vi "Render.vi"(8 "error in":errorcluster, 10 "Renderer in":refnum<class "Renderer.lvclass">, 11 "Dqmh Event in":refnum<class "Dqmh Event.lvclass">) -> (0 "error out":errorcluster, 3 "Sections out":refnum<class "Section.lvclass">[](array[class]))   [LabVIEW 2021, in "TAF Proj Document Type.lvlib" / "Dqmh Event.lvclass"]
uses:
  <vilib>/Wovalab/AntiDoc/Document Type/Add-ons/LabVIEW TAF Project/Dqmh Event/Dqmh Event.lvclass
  C:/Program Files (x86)/National Instruments/LabVIEW 2021/vi.lib/Wovalab/AntiDoc/Document Type/Add-ons/LabVIEW TAF Project/Vi/Vi.lvclass
  C:/Program Files (x86)/National Instruments/LabVIEW 2021/vi.lib/Wovalab/AntiDoc/Bloc/Bloc.lvclass
  <vilib>/Wovalab/AntiDoc/Renderer/Renderer.lvclass
  <vilib>/Wovalab/AsciiDoc for LabVIEW/Section/Section.lvclass
  <vilib>/Wovalab/AntiDoc/Document Type/Add-ons/LabVIEW TAF Project/Dqmh Event/Dqmh Event.lvclass/Dqmh Event.ctl
  <vilib>/Wovalab/AntiDoc/Document Type/Add-ons/LabVIEW TAF Project/Vi/Vi.lvclass/Vi.ctl
  <vilib>/Wovalab/AntiDoc/Bloc/Bloc.lvclass/Bloc.ctl
  <vilib>/Wovalab/AntiDoc/Renderer/Renderer.lvclass/Renderer.ctl
  <vilib>/Wovalab/AntiDoc/Renderer/Read Image Folder Path.vi
  <vilib>/Wovalab/AntiDoc/Document Type/Add-ons/LabVIEW TAF Project/Dqmh Event/Read Event Type.vi
  <vilib>/Wovalab/AntiDoc/Document Type/Add-ons/LabVIEW TAF Project/Vi/Read Conpane Image.vi
  <vilib>/Wovalab/AntiDoc/Bloc/Read Name.vi
  <vilib>/Wovalab/AntiDoc/Document Type/Add-ons/LabVIEW TAF Project/Vi/Read Description.vi
  <vilib>/Wovalab/AsciiDoc for LabVIEW/Paragraph/Paragraph.lvclass
  C:/Program Files (x86)/National Instruments/LabVIEW 2021/vi.lib/Wovalab/AsciiDoc for LabVIEW/Adoc-Bloc/Bloc.lvclass
  <vilib>/Wovalab/Asciidoc for LabVIEW/Image/Image.lvclass
  <vilib>/Wovalab/AsciiDoc for LabVIEW/Section/Add Bloc (array).vi
  <vilib>/Wovalab/AntiDoc/Document Type/Add-ons/LabVIEW TAF Project/TAF Proj Document Type.lvlib
  <vilib>/Wovalab/AntiDoc/Utilities/Utilities.lvlib
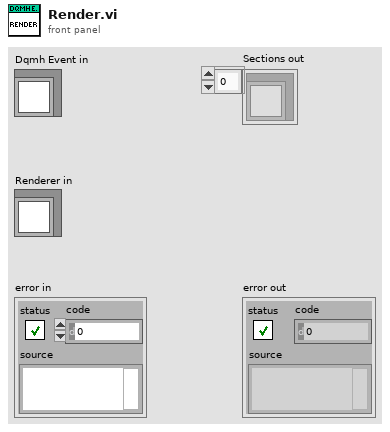
[diagram p1: front panel]
types:
  T1 = typedef "TAF Proj Document Type.lvlib/Project Parser.lvlib/Dqmh Event Type--enum.ctl" = enum16{"Not a DQMH Event", "Request", "Request And Wait For Reply", "Broadcast"}
  T2 = typedef "imagedata.ctl" = cluster{"image type":i32, "image depth":i32, "image":u8[], "mask":u8[], "colors":u32[], "Rectangle":cluster{"left":i16, "top":i16, "right":i16, "bottom":i16}}
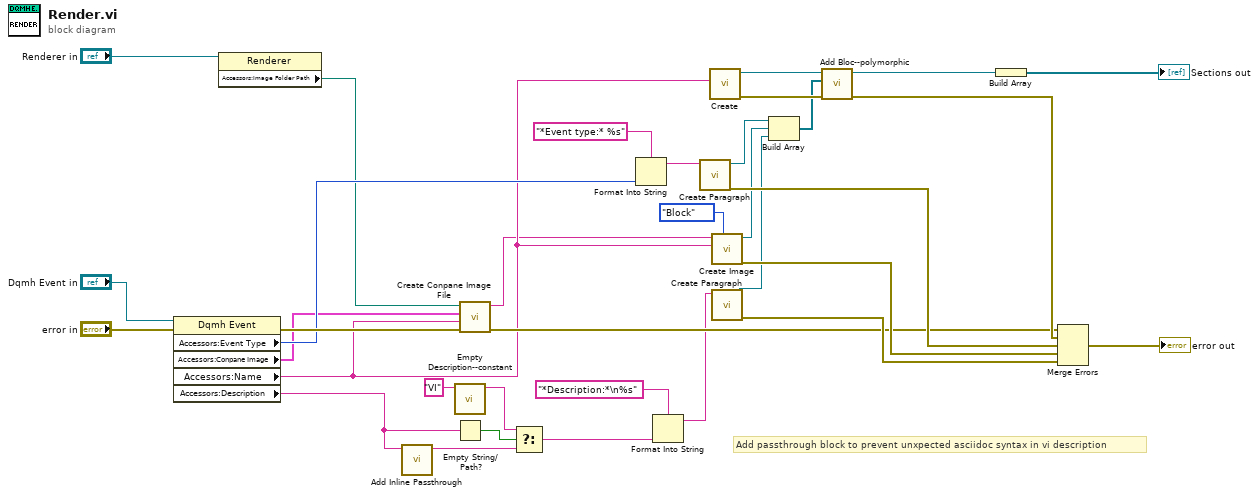
[diagram p0: block diagram]
diagram:
  # "Add passthrough block to prevent unxpected asciidoc syntax in vi description"
  n1 = property class="Dqmh Event"(reference="Dqmh Event in", error in="error in") -> (error out=w27:errorcluster, "Accessors:Event Type"=w15:T1, "Accessors:Conpane Image"=w9:T2, "Accessors:Name"=w8:string, "Accessors:Description"=w1:string)  [unwired: 1 out]
  n2 = property class="Renderer"(reference="Renderer in") -> ("Accessors:Image Folder Path"=w10:path)  [unwired: 1 in, 2 out]
  n3 = call <vilib>:"Add Inline Passthrough.vi"("String in"=w1) -> ("String out"=w2:string)  [unwired: 10 in]
  n4 = call <vilib>:"Empty Description--constant.vi"("Description Source"="VI") -> ("Empty Description"=w4:string)  [unwired: 10 in]
  n5 = Empty String/Path?(string/path=w1) -> (empty?=w18:bool)
  n6 = call <vilib>:"Create Conpane Image File.vi"("error in"=w27, "Name"=w8, "Conpane Image"=w9, "Image Folder Path"=w10) -> ("error out"=w26:errorcluster, "File Name"=w7:string)  [unwired: 6 in]
  n7 = Select(t=w4, s=w18, f=w2) -> (s? t:f=w11:string)
  n8 = Format Into String(format string="*Event type:* %s", w15) -> (resulting string=w17:string)  [unwired: 2 in, 1 out]
  n9 = Format Into String(format string="*Description:*\n%s", w11) -> (resulting string=w13:string)  [unwired: 2 in, 1 out]
  n10 = call <vilib>:"Create Paragraph.vi"("Content"=w17) -> ("error out"=w31:errorcluster, "Paragraph out"=w14:refnum<class "Paragraph.lvclass">)  [unwired: 9 in]
  n11 = call <vilib>:"Create.vi"("Title"=w8) -> ("error out"=w34:errorcluster, "Section out"=w23:refnum<class "Section.lvclass">)  [unwired: 9 in]
  n12 = call <vilib>:"Create Image.vi"("Type"=enum16{"Block", "Inline"}."Block", "Alt Text"=w8, "Image Path"=w7) -> ("error out"=w33:errorcluster, "Image out"=w20:refnum<class "Image.lvclass">)  [unwired: 7 in]
  n13 = call <vilib>:"Create Paragraph.vi"("Content"=w13) -> ("error out"=w32:errorcluster, "Paragraph out"=w22:refnum<class "Paragraph.lvclass">)  [unwired: 9 in]
  n14 = Build Array(w14, w20, w22) -> (w21:refnum<class "Bloc.lvclass">[])
  n15 = call-poly <vilib>:"Add Bloc--polymorphic.vi"("error in"=w34, "Bloc"=w21, "Section in"=w23) -> ("error out"=w28:errorcluster, "Section out"=w6:refnum<class "Section.lvclass">)  [unwired: 7 in]
  n16 = Build Array(w6) -> (→"Sections out":refnum<class "Section.lvclass">[])
  n17 = Merge Errors(w26, w28, w31, w33, w32) -> (→"error out":errorcluster)
